vi "Phasor Demo.vi"() -> ()   [LabVIEW 2020]
uses:
  <vilib>/Platform/TimedLoop/XDataNode/timing_clust.ctl
  <vilib>/Platform/TimedLoop/XDataNode/nitl_modes.ctl
  <vilib>/Platform/TimedLoop/XDataNode/wakeup.ctl
  <vilib>/Analysis/1siggen.llb/Ramp Pattern by Samples.vi
  <vilib>/platform/TimedLoop/XDataNode/XDataNode.xnode
  <vilib>/Analysis/NI_AALBase.lvlib
  <vilib>/Platform/TimedLoop/XDataNode/XDNodeRunTimeDep.lvlib
panel:
  out "Waveform Chart":waveform(dbl)[](graph)=[{"t0"=timestamp(3631171649.746716 s since 1904-01-01), "dt"=0.01, "Y"=[0.7289686274214104]}, {"t0"=timestamp(3631171649.746716 s since 1904-01-01), "dt"=0.01, "Y"=[0.6845471059286898]}]
  in  "Stop":bool
  in  "dt [s]":dbl=0.01 format="%#_13g"
  in  "f [Hz]":dbl=0.2 min=0.0 max=10.0 step=0.1 format="%#_13g"
  out "XY Graph":cluster{dbl[], dbl[]}[](graph)
  # "Phasor Demo"
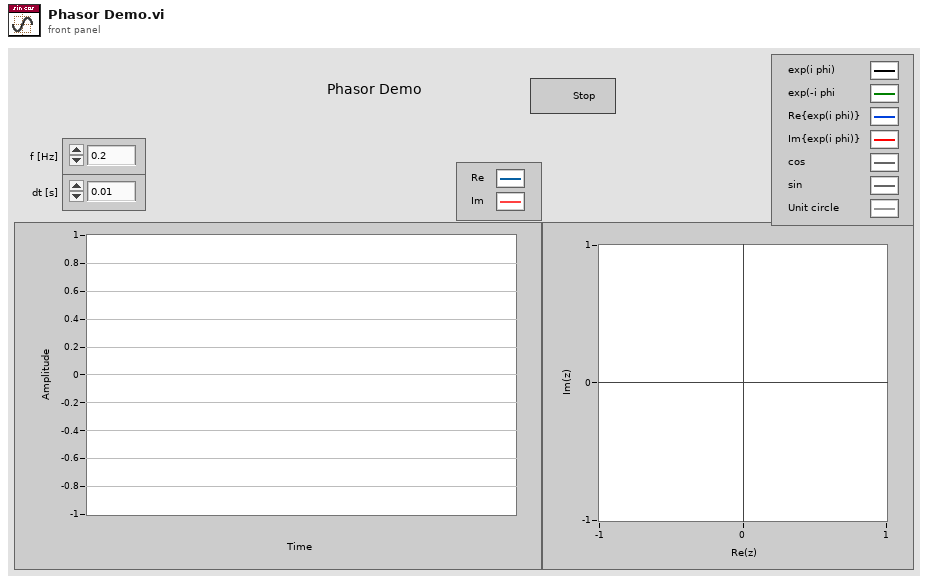
[diagram p1: front panel]
types:
  T1 = typedef "XDNodeRunTimeDep.lvlib/timing_clust.ctl" = cluster{"Expected End [f-1]":u64, "Actual End [f-1]":u64, "Finished Late? [f-1]":bool, "Expected End [i-1]":u64, "Actual End [i-1]":u64, "Finished Late? [i-1]":bool, "Expected Start [i]":u64, "Actual Start [i]":u64, "Expected Start [f]":u64, "Actual Start [f]":u64, "Source Name":string, "Structure Name":string, "Period":i64, "Deadline":i64, "Offset":i64, "Start":i64, "Priority":i32, "Timeout":i32, "Mode":T2, "Wakeup Reason":T3, "Error":errorcluster, "Source Type":string, "Secondary Source Type":string, "Global End Time":u64, "Global Start Time":u64, "Frame Duration":u64, "Iteration Duration":u64, "Assigned CPU":i32, "I/O Scan Engine Mode":u32}
  T2 = typedef "XDNodeRunTimeDep.lvlib/nitl_modes.ctl" = enum32{"No Change", "Process missed periods, maintain original phase", "Discard missed periods, maintain original phase", "Process missed periods, ignore original phase", "Discard missed periods, ignore original phase"}
  T3 = typedef "XDNodeRunTimeDep.lvlib/wakeup.ctl" = enum32{"Normal", "Aborted", "Asynchronous wakeup", "Timing source error", "Timed loop error", "Timeout"}
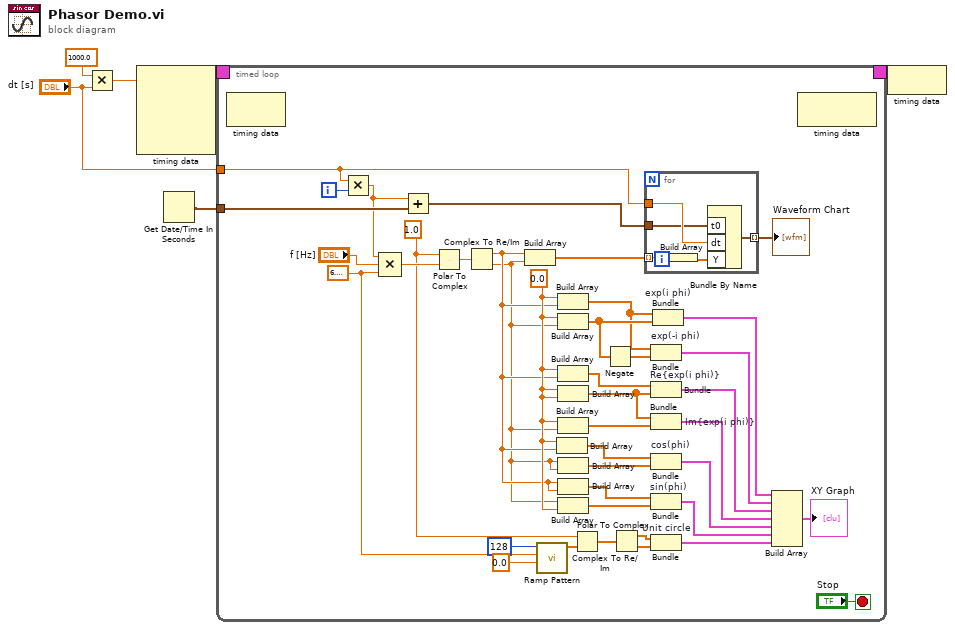
[diagram p0: block diagram]
diagram:
  n1 = Multiply(x=1000.0, y="dt [s]") -> (x*y=w3:dbl)
  n2 = node-c288(w3) -> (w6:T1)  [unwired: 3 in]
  n3 = Get Date/Time In Seconds() -> (seconds since 1Jan1904=w1:timestamp)
  n4 = timed-loop {
    timing: w6 -> [_]
    timing-out: [_] -> w5
    tunnel: "dt [s]" -> [w10]
    tunnel: w1 -> [w9]
    i -> [w43]
    stop <- "Stop" stop-if-true
    w17 = 0.0 ("r")
    w34 = 1.0 ("r")
    w12 = 6.283185307179586
    n5 = node-c288() -> ()  [unwired: 1 in, 1 out]
    n6 = Multiply(x=w10, y=w43) -> (x*y=w8:dbl)
    n7 = Compound Arithmetic op=MULTIPLY(w8, "f [Hz]", w12) -> (w45:dbl)
    n8 = Add(x=w8, y=w9) -> (x+y=w7:timestamp)
    n9 = Polar To Complex(1:w45, 2:w34) -> (0:w42:cdb)
    n10 = Complex To Re/Im(x + iy=w42) -> (x=w15:dbl, y=w14:dbl)
    n11 = Build Array(w15, w14) -> (w13:dbl[])
    n12 = call-poly <vilib>:"Ramp Pattern.vi"("start"=0.0, "end"=w12, "samples"=128) -> ("Ramp Pattern"=w31:dbl[])  [unwired: 7 in, 1 out]
    n13 = Build Array(w17, w15) -> (w16:dbl[])
    n14 = Build Array(w17, w15) -> (w28:dbl[])
    n15 = Build Array(w17, w14) -> (w39:dbl[])
    n16 = Build Array(w17, w15) -> (w27:dbl[])
    n17 = Build Array(w17, w17) -> (w22:dbl[])
    n18 = Build Array(w17, w14) -> (w20:dbl[])
    n19 = Build Array(w14, w14) -> (w18:dbl[])
    n20 = Build Array(w15, w15) -> (w26:dbl[])
    n21 = Build Array(w14, w17) -> (w25:dbl[])
    n22 = Polar To Complex(1:w31, 2:w34) -> (0:w35:cdb[])
    n23 = Negate(x=w39) -> (-x=w38:dbl[])
    n24 = Complex To Re/Im(x + iy=w35) -> (x=w30:dbl[], y=w29:dbl[])
    n25 = for {
      tunnel: w13 -> [w51] mode=indexing
      tunnel: w10 -> [w49]
      tunnel: [w48] -> w11 mode=indexing
      tunnel: w7 -> [w47]
      n26 = Build Array(w51) -> (w50:dbl[])
      n27 = Bundle By Name("t0"=w47, "dt"=w49, "Y"=w50) -> (w48:waveform(dbl))  [unwired: 1 in]
    }
    "Waveform Chart" <- w11
    n28 = Bundle "exp(-i phi)"(w28, w38) -> (w36:cluster{dbl[], dbl[]})  [unwired: 1 in]
    n29 = Bundle "Re{exp(i phi)}"(w27, w22) -> (w40:cluster{dbl[], dbl[]})  [unwired: 1 in]
    n30 = Bundle "Im{exp(i phi)}"(w22, w20) -> (w21:cluster{dbl[], dbl[]})  [unwired: 1 in]
    n31 = Bundle "cos(phi)"(w16, w18) -> (w19:cluster{dbl[], dbl[]})  [unwired: 1 in]
    n32 = Bundle "sin(phi)"(w26, w25) -> (w23:cluster{dbl[], dbl[]})  [unwired: 1 in]
    n33 = Bundle "Unit circle"(w30, w29) -> (w24:cluster{dbl[], dbl[]})  [unwired: 1 in]
    n34 = Bundle "exp(i phi)"(w28, w39) -> (w37:cluster{dbl[], dbl[]})  [unwired: 1 in]
    n35 = Build Array(w37, w36, w40, w21, w19, w23, w24) -> (→"XY Graph":cluster{dbl[], dbl[]}[])
    n36 = node-c288() -> ()  [unwired: 1 in, 1 out]
  }
  n37 = node-c288(w5) -> ()
